vi "HandleError.vi"(8 "ErrorArray":errorcluster[](array[cluster])) -> (0 "ErrorArray":errorcluster[](array[cluster]), 2 "XML_Out":string[](array[string]), 4 "Stop":bool)   [LabVIEW 2014, in "Test.lvclass"]
uses:
  Test.lvclass
  Queue/clQueMsgType.ctl
  <vilib>/Utility/error.llb/Error Cluster From Error Code.vi
  <vilib>/ErrorRing/Error Ring.xnode
  <userlib>/NIST/NISTErrorLib/NISTErrorLib.lvlib
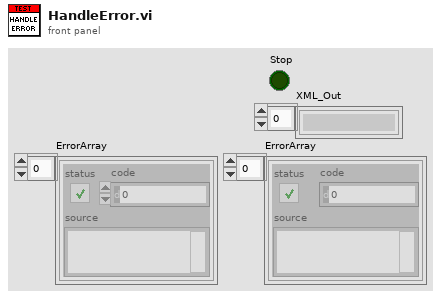
[diagram p1: front panel]
types:
  T1 = typedef "Test.lvclass/clQueMsgType.ctl" = cluster{"Message":string, "Data":variant}
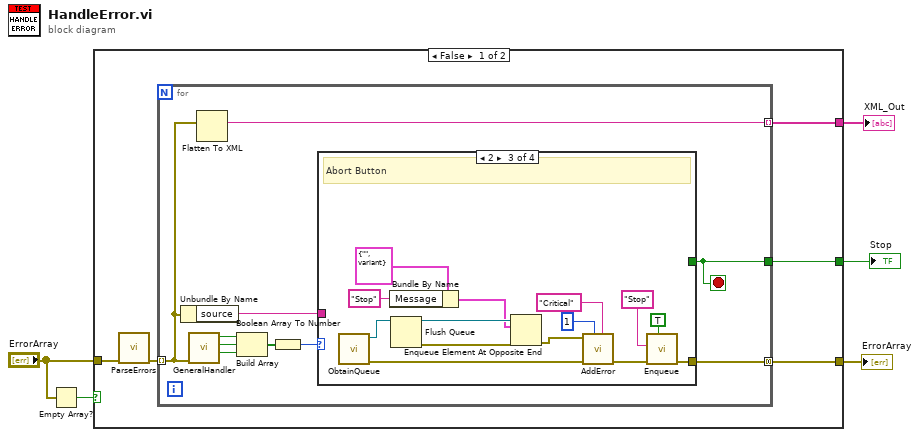
[diagram p0: block diagram]
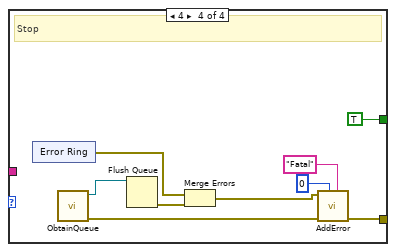
[diagram p5: hidden frame]
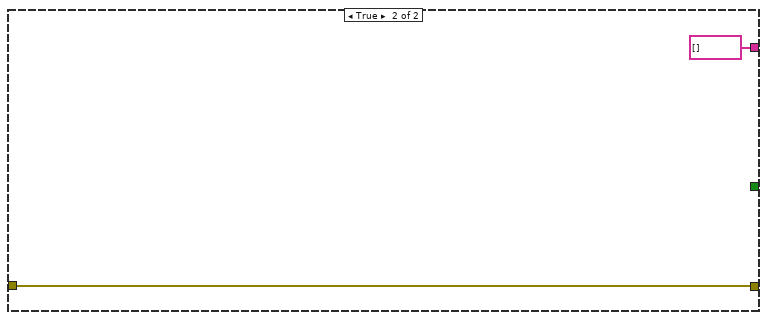
[diagram p6: hidden frame]
diagram:
  n1 = Empty Array?(array="ErrorArray") -> (empty?=w5:bool)
  n2 = case shown="False" w5 {
    tunnel: [w7 w51] -> w3
    tunnel: "ErrorArray" -> [w10 w51]
    tunnel: [w8 string[] []] -> w2
    tunnel: [w6 _] -> w1
    frame False {
      n3 = call <userlib>:"ParseErrors.vi"("ErrorArray"=w10) -> ("ErrorArray"=w9:errorcluster[])  [unwired: 8 in, 2 out]
      n4 = for {
        tunnel: w9 -> [w20] mode=indexing
        tunnel: [w19] -> w8 mode=indexing
        tunnel: [w12] -> w7 mode=concatenating
        tunnel: [w11] -> w6
        stop <- w11 stop-if-true
        n5 = Unbundle By Name(w20) -> ("source"=w13:string)
        n6 = call <userlib>:"GeneralHandler.vi"("error in (no error)"=w20) -> ("Stop"=w16:bool, "Abort"=w17:bool, "Continue"=w18:bool)  [unwired: 7 in, 1 out]
        n7 = Flatten To XML(anything=w20) -> (xml string=w19:string)
        n8 = Build Array(w18, w17, w16) -> (w15:bool[])
        n9 = Boolean Array To Number(Boolean array=w15) -> (number=w14:u32)
        n10 = case shown="2" w14 {
          tunnel: w13 -> [_ w21 _ _]
          tunnel: [_ _ w25 w40] -> w12
          tunnel: [_ _ _ TRUE] -> w11
          frame 0, Default {
            # "No Dialog"
          }
          frame 1 {
            # "Continue"
            n11 = case shown="\"Log\"" w21 {
              frame "False", Default {
              }
              frame "Log" {
                # "TODO:  Add Logging"
              }
            }
          }
          frame 2 {
            # "Abort Button"
            n12 = call "ObtainQueue.vi"() -> ("ErrorArray."=w29:errorcluster[], "TstQue"=w35:refnum<queue>)  [unwired: 10 in]
            n13 = Bundle By Name(cluster=T1 {"Message"="", "Data"=variant} ("clQueMsgType"), "Message"="Stop") -> (w30:T1)
            n14 = Flush Queue(queue=w35) -> (queue out=w33:refnum<queue>, error out=w34:errorcluster)  [unwired: 1 in, 1 out]
            n15 = Enqueue Element At Opposite End(queue=w33, element=w30, error in (no error)=w34) -> (error out=w28:errorcluster)  [unwired: 1 in, 2 out]
            n16 = call <userlib>:"AddError.vi"("Severity"="Critical", "Priority"=u8 1, "ErrorArray"=w29, "error in (no error)"=w28) -> ("ErrorArray"=w24:errorcluster[])  [unwired: 6 in, 1 out]
            n17 = call "Enqueue.vi"("Priority? (f)"=TRUE, "ErrorArray"=w24, "Message"="Stop") -> ("ErrorArray"=w25:errorcluster[])  [unwired: 8 in]
          }
          frame 4 {
            # "Stop"
            n18 = xnode "Error Ring"() -> ("error out"=w41:errorcluster)
            n19 = call "ObtainQueue.vi"() -> ("ErrorArray."=w36:errorcluster[], "TstQue"=w42:refnum<queue>)  [unwired: 10 in]
            n20 = Flush Queue(queue=w42) -> (error out=w43:errorcluster)  [unwired: 1 in, 2 out]
            n21 = Merge Errors(w41, w43) -> (w37:errorcluster)
            n22 = call <userlib>:"AddError.vi"("Severity"="Fatal", "Priority"=u8 0, "ErrorArray"=w36, "error in (no error)"=w37) -> ("ErrorArray"=w40:errorcluster[])  [unwired: 6 in, 1 out]
          }
        }
      }
    }
    frame True {
    }
  }
  "ErrorArray" <- w3
  "Stop" <- w1
  "XML_Out" <- w2
